vi "LargeFolder_TO_Pointcloud.vi"() -> ()   [LabVIEW 2016]
panel:
  in  "Large Sweep Folder":path=path "B:/SketchSET/SA03008H.20180718/77_B+SG_B_-7to0inc1_SG_-0.5to0.5inc0.25_at0.2Hz_-300mVto-100mV_IV_@BG15"
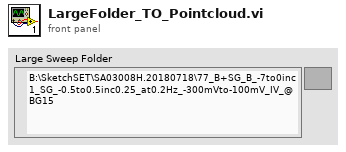
[diagram p1: front panel]
types:
  T1 = cluster{"upper limit":dbl, dbl, "upper limit":dbl, "upper limit":dbl}
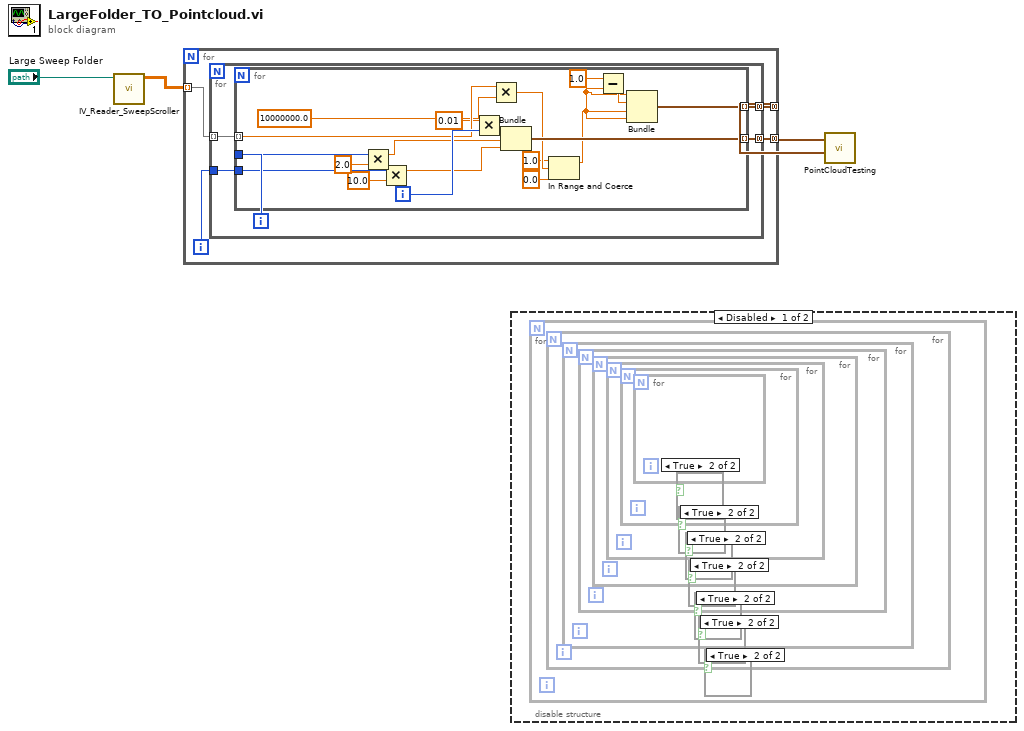
[diagram p0: block diagram]
diagram:
  n1 = call "IV_Reader_SweepScroller.vi"("Large Sweep Folder"="Large Sweep Folder") -> ("Arr_Of_IV_Intensites"=w3:dbl[][][])  [unwired: 10 in]
  n2 = for {
    tunnel: w3 -> [w8] mode=indexing
    tunnel: [w6] -> w2 mode=concatenating
    tunnel: [w5] -> w1 mode=concatenating
    i -> [w7]
    n3 = for {
      tunnel: w8 -> [w13] mode=indexing
      tunnel: w7 -> [w11]
      tunnel: [w10] -> w6 mode=concatenating
      tunnel: [w9] -> w5 mode=concatenating
      i -> [w12]
      n4 = for {
        tunnel: w13 -> [w28] mode=indexing
        tunnel: w12 -> [w32]
        tunnel: w11 -> [w31]
        tunnel: [w30] -> w10 mode=indexing
        tunnel: [w26] -> w9 mode=indexing
        i -> [w29]
        n5 = Multiply(x=w32, y=2.0) -> (x*y=w20:dbl)
        n6 = Multiply(x=w31, y=10.0) -> (x*y=w18:dbl)
        n7 = Multiply(x=0.01, y=w29) -> (x*y=w22:dbl)
        n8 = Multiply(x=w28, y=10000000.0) -> (x*y=w25:dbl)
        n9 = Bundle(w22, w20, w18) -> (w30:cluster{dbl, dbl, dbl})  [unwired: 1 in]
        n10 = In Range and Coerce(upper limit=1.0, x=w25, lower limit=0.0) -> (coerced(x)=w15:dbl)  [unwired: 1 out]
        n11 = Subtract(x=1.0, y=w15) -> (x-y=w16:dbl)
        n12 = Bundle("upper limit"=w15, w16, "upper limit"=w15, "upper limit"=w15) -> (w26:T1)  [unwired: 1 in]
      }
    }
  }
  n13 = disable-structure shown="Disabled" {
    frame Disabled {
      n14 = for {
        n15 = for {
          n16 = for {
            n17 = for {
              n18 = for {
                n19 = for {
                  n20 = for {
                    n21 = for {
                    }
                    n22 = case shown="True" {
                      selector: _ -> [_ _]
                      frame False {
                      }
                      frame True {
                      }
                    }
                  }
                  n23 = case shown="True" {
                    selector: _ -> [_ _]
                    frame False {
                    }
                    frame True {
                    }
                  }
                }
                n24 = case shown="True" {
                  selector: _ -> [_ _]
                  frame False {
                  }
                  frame True {
                  }
                }
              }
              n25 = case shown="True" {
                selector: _ -> [_ _]
                frame False {
                }
                frame True {
                }
              }
            }
            n26 = case shown="True" {
              selector: _ -> [_ _]
              frame False {
              }
              frame True {
              }
            }
          }
          n27 = case shown="True" {
            selector: _ -> [_ _]
            frame False {
            }
            frame True {
            }
          }
        }
        n28 = case shown="True" {
          selector: _ -> [_ _]
          frame False {
          }
          frame True {
          }
        }
      }
    }
    frame Enabled {
    }
  }
  n29 = call "PointCloudTesting.vi"("Array"=w1, "Array of Vertices"=w2) -> ()  [unwired: 10 in]
